vi "Press_Calc.vi"(7 "tfine":dbl, 10 "PressCoeff":T1, 11 "PressureReadingU32":u32) -> (2 "Pressure(Pa)":dbl)   [LabVIEW 2020, in "BMP208.lvclass"]
uses:
  BMP208.lvclass
  Controls/td_cluster_Press_Coeff.ctl
panel:
  out "PressureReadingU32 2":u32 format="%020b"
  out "press(3)":dbl format="%9.2f"
  out "var2(4)":dbl
  out "var1(4)":dbl
  out "press(2)":dbl
  out "press(1)":dbl
  out "var1(3)":dbl
  out "var1(2)":dbl
  out "var2(3)":dbl format="%#_6f"
  out "var2(2)":dbl
  out "var2(1)":dbl
  out "var1":dbl
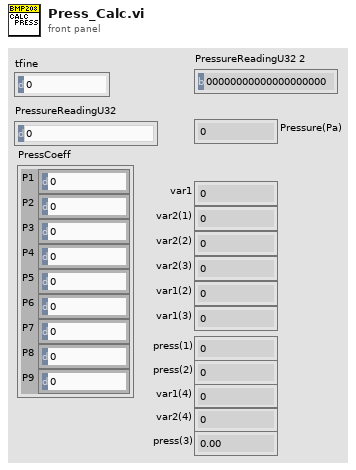
[diagram p1: front panel]
types:
  T1 = typedef "BMP208.lvclass/td_cluster_Press_Coeff.ctl" = cluster{"P1":u16, "P2":i16, "P3":i16, "P4":i16, "P5":i16, "P6":i16, "P7":i16, "P8":i16, "P9":i16}
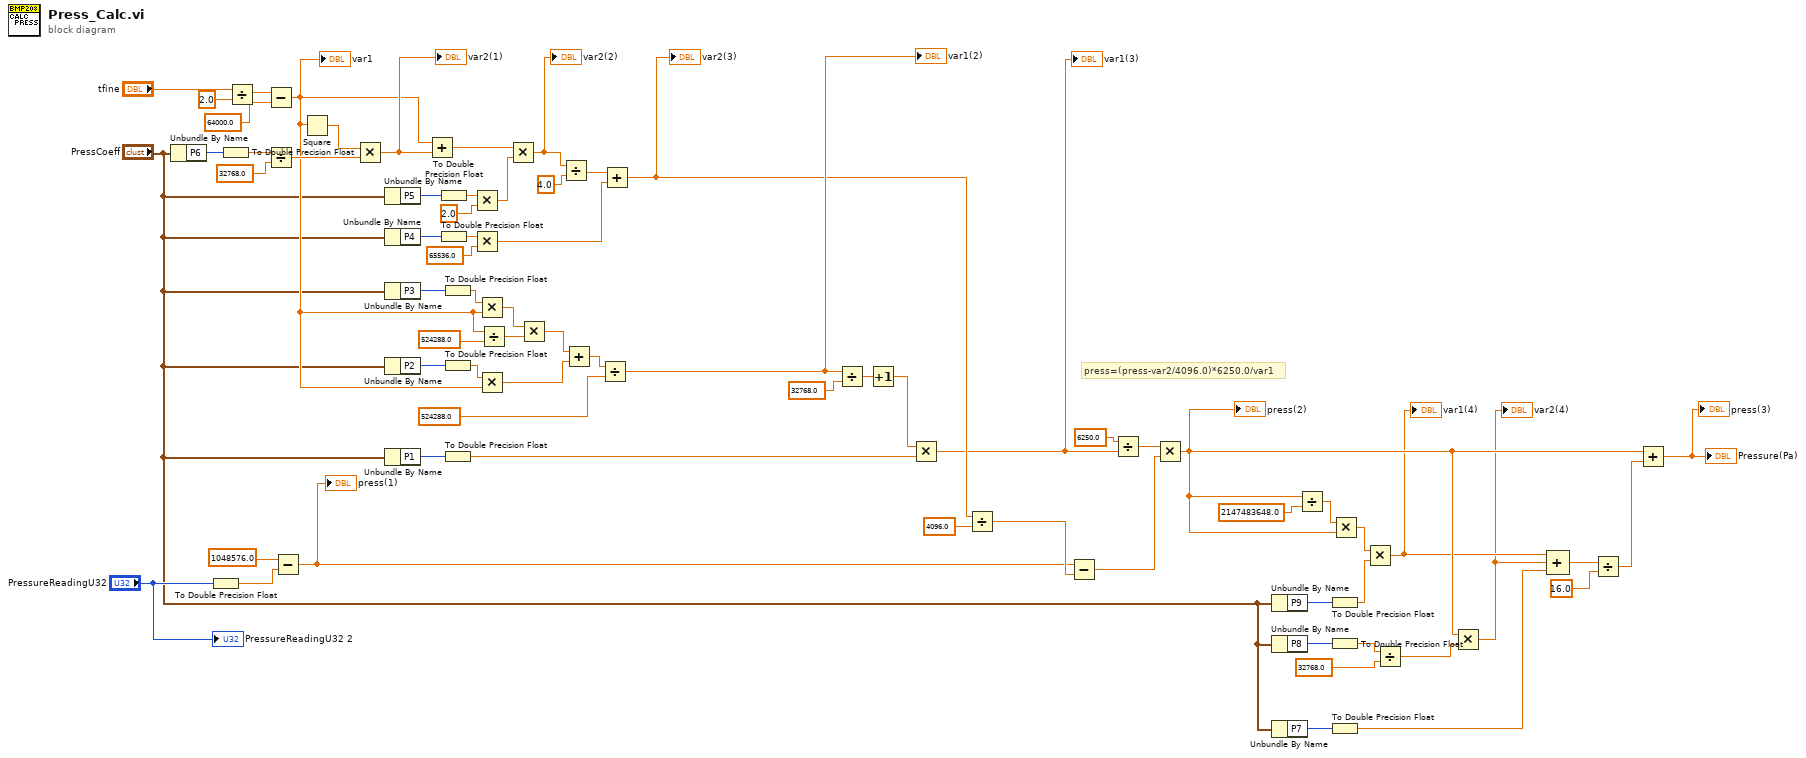
[diagram p0: block diagram]
diagram:
  # "press=(press-var2/4096.0)*6250.0/var1"
  n1 = Unbundle By Name("PressCoeff") -> ("P6"=w66:i16)
  n2 = To Double Precision Float(number="PressureReadingU32") -> (double precision float=w28:dbl)
  n3 = To Double Precision Float(number=w66) -> (double precision float=w65:dbl)
  n4 = Divide(x="tfine", y=2.0) -> (x/y=w68:dbl)
  n5 = Subtract(x=w68, y=64000.0) -> (x-y=w40:dbl)
  "var1" <- w40
  n6 = Divide(x=w65, y=32768.0) -> (x/y=w64:dbl)
  n7 = Subtract(x=1048576.0, y=w28) -> (x-y=w24:dbl)
  "press(1)" <- w24
  n8 = Square(x=w40) -> (x^2=w48:dbl)
  n9 = Multiply(x=w48, y=w64) -> (x*y=w62:dbl)
  "var2(1)" <- w62
  n10 = Unbundle By Name("PressCoeff") -> ("P5"=w61:i16)
  n11 = Unbundle By Name("PressCoeff") -> ("P4"=w51:i16)
  n12 = Unbundle By Name("PressCoeff") -> ("P3"=w49:i16)
  n13 = Unbundle By Name("PressCoeff") -> ("P2"=w42:i16)
  n14 = Unbundle By Name("PressCoeff") -> ("P1"=w35:u16)
  n15 = Add(x=w40, y=w62) -> (x+y=w57:dbl)
  n16 = To Double Precision Float(number=w61) -> (double precision float=w59:dbl)
  n17 = To Double Precision Float(number=w51) -> (double precision float=w53:dbl)
  n18 = To Double Precision Float(number=w49) -> (double precision float=w47:dbl)
  n19 = To Double Precision Float(number=w42) -> (double precision float=w41:dbl)
  n20 = To Double Precision Float(number=w35) -> (double precision float=w36:dbl)
  n21 = Multiply(x=w59, y=2.0) -> (x*y=w58:dbl)
  n22 = Multiply(x=w53, y=65536.0) -> (x*y=w50:dbl)
  n23 = Multiply(x=w47, y=w40) -> (x*y=w45:dbl)
  n24 = Multiply(x=w41, y=w40) -> (x*y=w39:dbl)
  n25 = Divide(x=w40, y=524288.0) -> (x/y=w44:dbl)
  n26 = Multiply(x=w57, y=w58) -> (x*y=w56:dbl)
  "var2(2)" <- w56
  n27 = Multiply(x=w45, y=w44) -> (x*y=w43:dbl)
  n28 = Divide(x=w56, y=4.0) -> (x/y=w54:dbl)
  n29 = Add(x=w43, y=w39) -> (x+y=w38:dbl)
  n30 = Divide(x=w38, y=524288.0) -> (x/y=w32:dbl)
  "var1(2)" <- w32
  n31 = Add(x=w54, y=w50) -> (x+y=w27:dbl)
  "var2(3)" <- w27
  n32 = Divide(x=w32, y=32768.0) -> (x/y=w34:dbl)
  n33 = Increment(x=w34) -> (x+1=w31:dbl)
  n34 = Multiply(x=w31, y=w36) -> (x*y=w22:dbl)
  "var1(3)" <- w22
  n35 = Divide(x=w27, y=4096.0) -> (x/y=w25:dbl)
  n36 = Subtract(x=w24, y=w25) -> (x-y=w20:dbl)
  n37 = Divide(x=6250.0, y=w22) -> (x/y=w21:dbl)
  n38 = Multiply(x=w21, y=w20) -> (x*y=w10:dbl)
  "press(2)" <- w10
  n39 = Unbundle By Name("PressCoeff") -> ("P9"=w18:i16)
  n40 = Unbundle By Name("PressCoeff") -> ("P8"=w14:i16)
  n41 = Unbundle By Name("PressCoeff") -> ("P7"=w8:i16)
  n42 = Divide(x=w10, y=2147483648.0) -> (x/y=w16:dbl)
  n43 = To Double Precision Float(number=w18) -> (double precision float=w19:dbl)
  n44 = To Double Precision Float(number=w14) -> (double precision float=w13:dbl)
  n45 = To Double Precision Float(number=w8) -> (double precision float=w5:dbl)
  n46 = Multiply(x=w16, y=w10) -> (x*y=w15:dbl)
  n47 = Multiply(x=w15, y=w19) -> (x*y=w7:dbl)
  "var1(4)" <- w7
  n48 = Divide(x=w13, y=32768.0) -> (x/y=w11:dbl)
  n49 = Multiply(x=w10, y=w11) -> (x*y=w6:dbl)
  "var2(4)" <- w6
  n50 = Compound Arithmetic op=ADD(w7, w6, w5) -> (w4:dbl)
  n51 = Divide(x=w4, y=16.0) -> (x/y=w2:dbl)
  n52 = Add(x=w10, y=w2) -> (x+y=→"Pressure(Pa)" →"press(3)":dbl)
  "PressureReadingU32 2" <- "PressureReadingU32"
